vi "IsoSPI without MCU Spying Tool IHM.vi"() -> ()   [LabVIEW 2020]
uses:
  <vilib>/Instr/_visa.llb/VISA Flush IO Buffer Mask.ctl
  <vilib>/Utility/config.llb/Read Key (Double).vi
  Variables globales outil isospi sans MCU.vi
  <vilib>/Utility/config.llb/Read Key (U32).vi
  <vilib>/Instr/_visa.llb/VISA Configure Serial Port (Instr).vi
  <vilib>/Utility/config.llb/NI_LVConfig.lvlib
panel:
  in  "stop":bool
  out "SumOfCellsVoltage":string[][](table)
  out "LTC6811 Temperatures":string[][](table)
  out "NTC Temperatures":string[][](table)
  out "Cell Voltages":string[][](table)
  out "String from arduino":string
  in  "VISA resource 2":refnum<visa-resource-name>
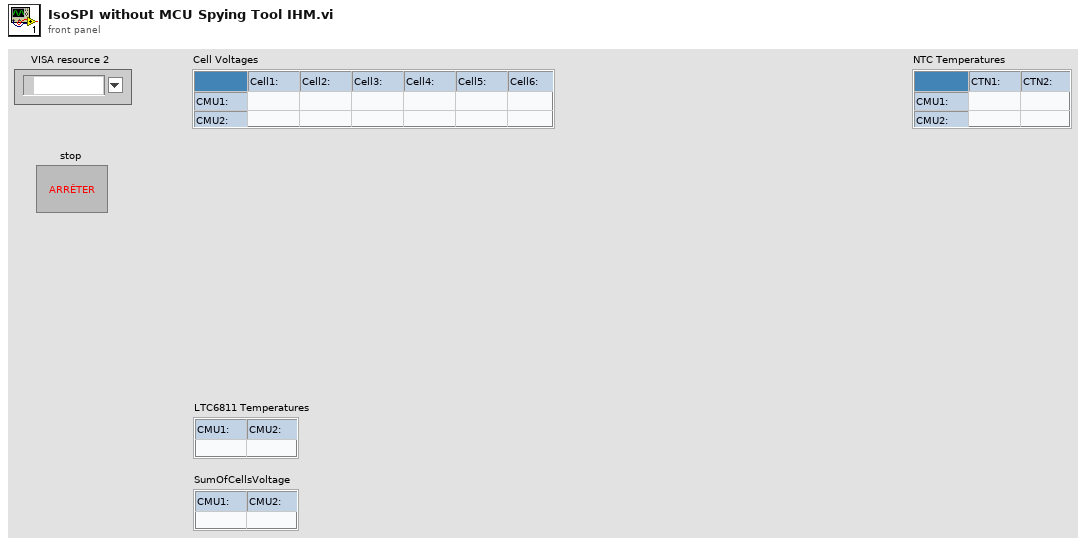
[diagram p1: front panel]
types:
  T1 = typedef "NI_LVConfig.lvlib/Config Data RefNum.ctl" = refnum<k1>
  T2 = typedef "VISA Flush IO Buffer Mask.ctl" = u16
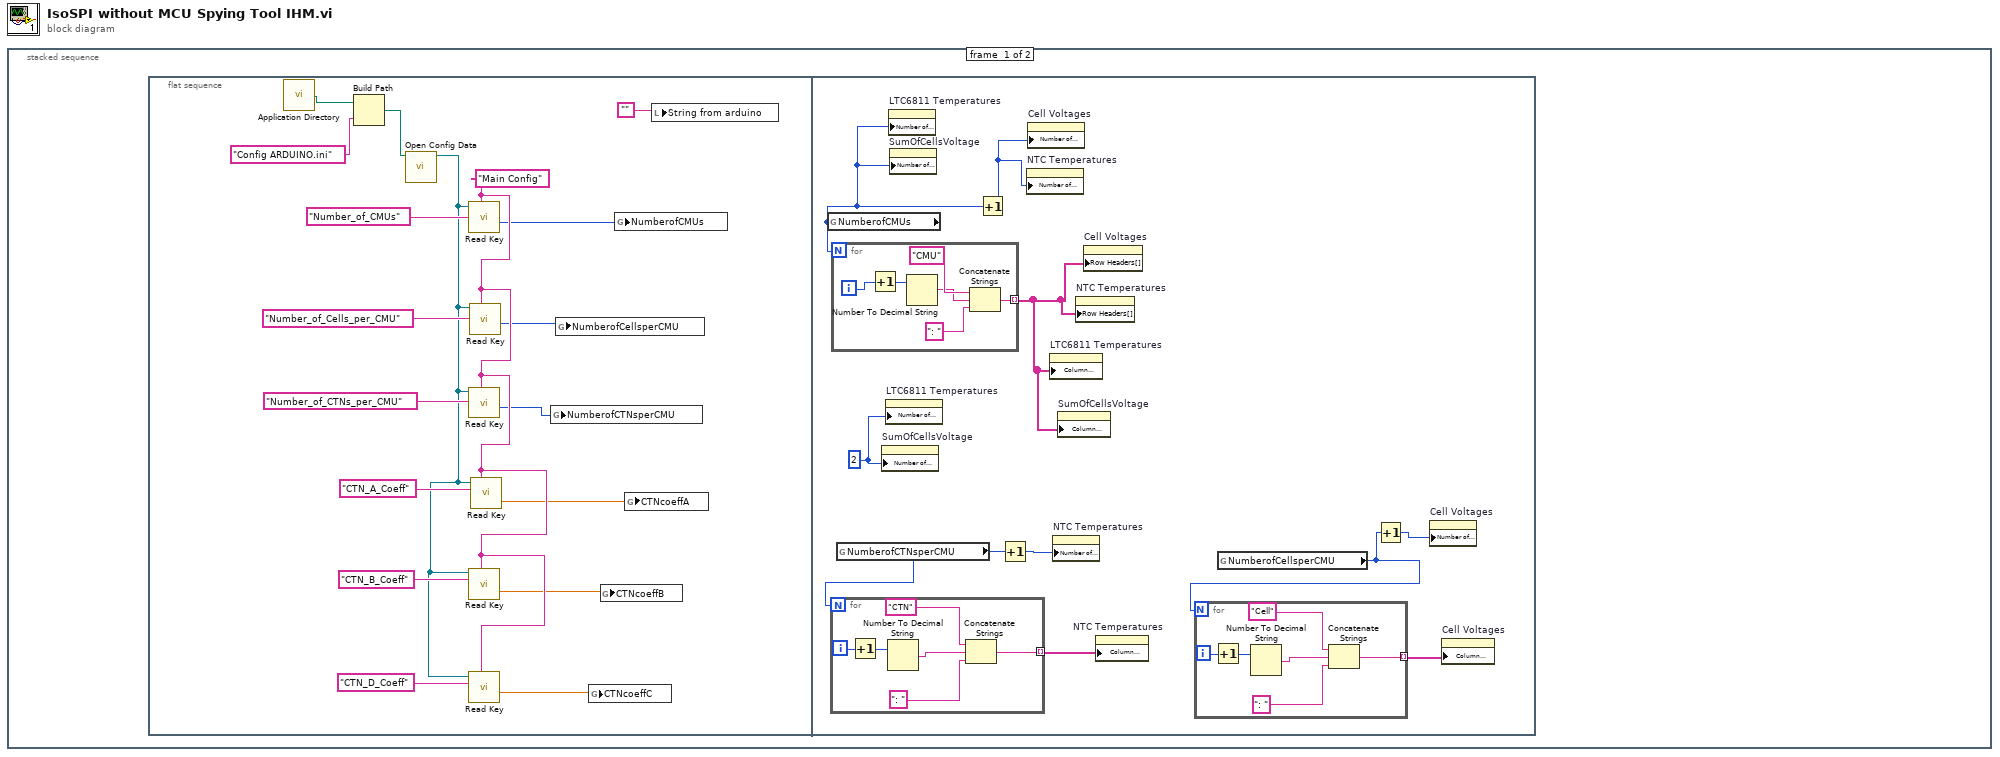
[diagram p0: block diagram]
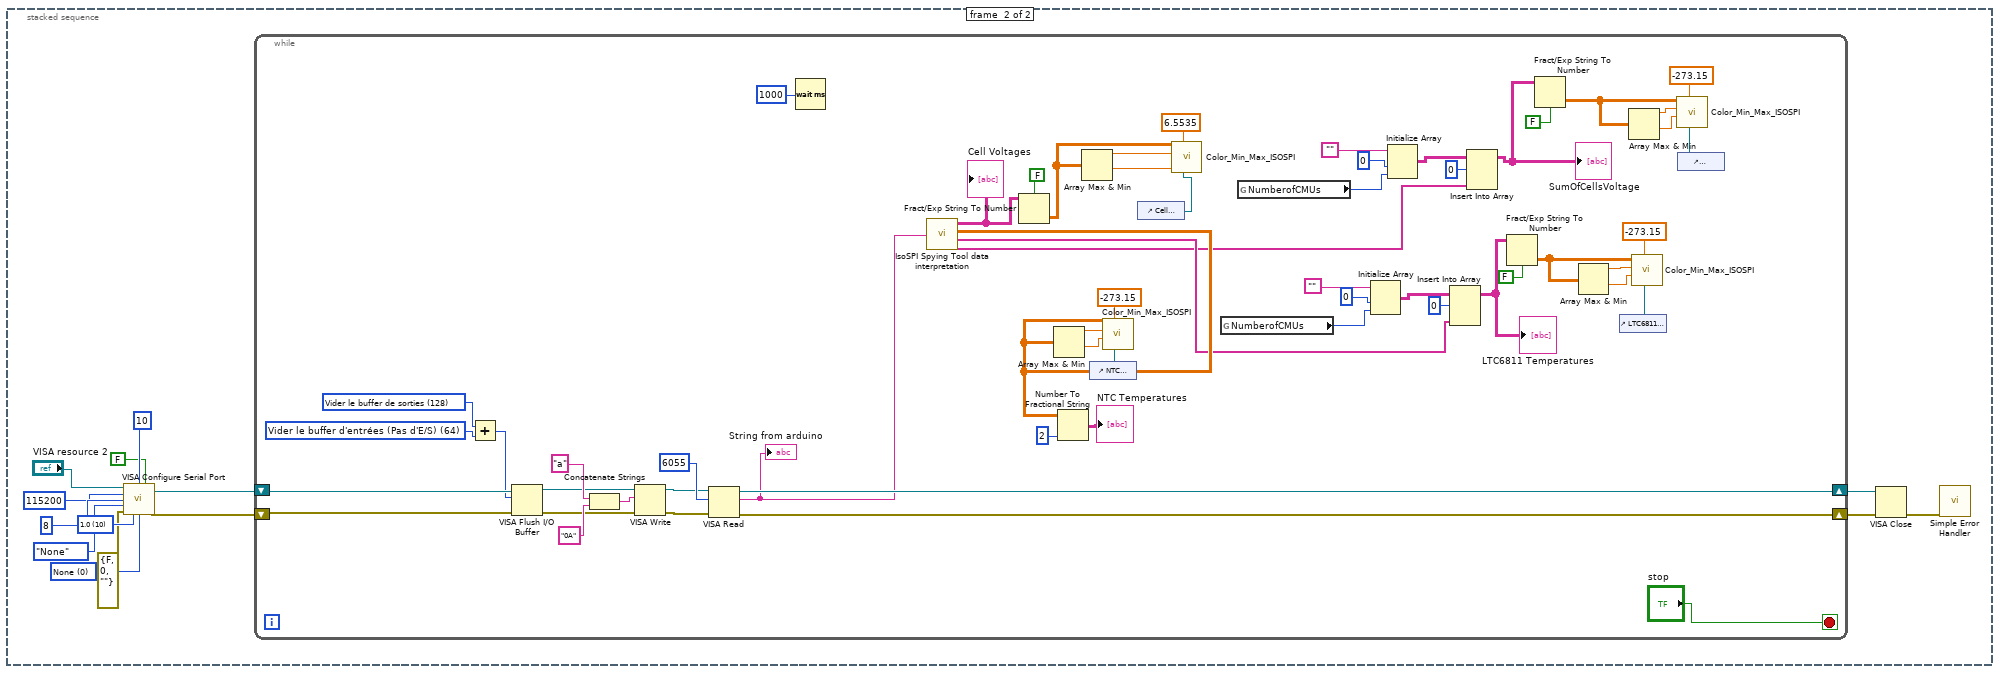
[diagram p2: hidden frame]
diagram:
  n1 = stacked-sequence {
    frame #0 {
      n2 = flat-sequence {
        frame #0 {
          w8 = "Main Config" ("section")
          n3 = call <vilib>:"Application Directory.vi"() -> ("Application Directory"=w18:path)
          n4 = Build Path(base path=w18, name or relative path="Config ARDUINO.ini") -> (appended path=w16:path)
          n5 = call <vilib>:"Open Config Data.vi"("configuration file path"=w16) -> ("refnum"=w9:T1)  [unwired: 8 in, 2 out]
          n6 = call-poly <vilib>:"Read Key.vi"("section"=w8, "key"="Number_of_CMUs", "refnum"=w9) -> ("value"=w7:u32)  [unwired: 5 in, 3 out]
          n7 = call-poly <vilib>:"Read Key.vi"("section"=w8, "key"="Number_of_CTNs_per_CMU", "refnum"=w9) -> ("value"=w5:u32)  [unwired: 5 in, 3 out]
          n8 = call-poly <vilib>:"Read Key.vi"("section"=w8, "key"="CTN_B_Coeff", "refnum"=w9) -> ("value"=w3:dbl)  [unwired: 5 in, 3 out]
          n9 = call-poly <vilib>:"Read Key.vi"("section"=w8, "key"="CTN_D_Coeff", "refnum"=w9) -> ("value"=w2:dbl)  [unwired: 5 in, 3 out]
          n10 = call-poly <vilib>:"Read Key.vi"("section"=w8, "key"="Number_of_Cells_per_CMU", "refnum"=w9) -> ("value"=w6:u32)  [unwired: 5 in, 3 out]
          n11 = call-poly <vilib>:"Read Key.vi"("section"=w8, "key"="CTN_A_Coeff", "refnum"=w9) -> ("value"=w4:dbl)  [unwired: 5 in, 3 out]
          n12 = global write "Variables globales outil isospi sans MCU.vi" "NumberofCTNsperCMU"(w5) -> ()
          n13 = global write "Variables globales outil isospi sans MCU.vi" "NumberofCellsperCMU"(w6) -> ()
          n14 = global write "Variables globales outil isospi sans MCU.vi" "CTNcoeffC"(w2) -> ()
          n15 = global write "Variables globales outil isospi sans MCU.vi" "CTNcoeffB"(w3) -> ()
          n16 = global write "Variables globales outil isospi sans MCU.vi" "NumberofCMUs"(w7) -> ()
          n17 = global write "Variables globales outil isospi sans MCU.vi" "CTNcoeffA"(w4) -> ()
          n18 = local write "String from arduino"("") -> ()
        }
        frame #1 {
          w20 = u32 2 ("Nombre de lignes")
          n19 = global read "Variables globales outil isospi sans MCU.vi" "NumberofCMUs"() -> (w19:u32)
          n20 = for {
            N: w19 -> [_]
            tunnel: [w41] -> w21 mode=indexing
            i -> [w46]
            n21 = Increment(x=w46) -> (x+1=w45:i32)
            n22 = Number To Decimal String(number=w45) -> (decimal integer string=w43:string)  [unwired: 1 in]
            n23 = Concatenate Strings("CMU", w43, ": ") -> (w41:string)
          }
          n24 = global read "Variables globales outil isospi sans MCU.vi" "NumberofCTNsperCMU"() -> (w24:u32)
          n25 = for {
            N: w24 -> [_]
            tunnel: [w29] -> w23 mode=indexing
            i -> [w34]
            n26 = Increment(x=w34) -> (x+1=w33:i32)
            n27 = Number To Decimal String(number=w33) -> (decimal integer string=w32:string)  [unwired: 1 in]
            n28 = Concatenate Strings("CTN", w32, ": ") -> (w29:string)
          }
          n29 = property on="SumOfCellsVoltage" class="Tbl (strict)"("Number of Rows"=w20) -> ()  [unwired: 2 in, 2 out]
          n30 = property on="LTC6811 Temperatures" class="Tbl (strict)"("Number of Rows"=w20) -> ()  [unwired: 2 in, 2 out]
          n31 = property on="LTC6811 Temperatures" class="Tbl (strict)"("Number of Columns"=w19) -> ()  [unwired: 2 in, 2 out]
          n32 = property on="SumOfCellsVoltage" class="Tbl (strict)"("Number of Columns"=w19) -> ()  [unwired: 2 in, 2 out]
          n33 = Increment(x=w19) -> (x+1=w22:u32)
          n34 = Increment(x=w24) -> (x+1=w25:u32)
          n35 = property on="NTC Temperatures" class="Tbl (strict)"("Number of Rows"=w22) -> ()  [unwired: 2 in, 2 out]
          n36 = property on="Cell Voltages" class="Tbl (strict)"("Number of Rows"=w22) -> ()  [unwired: 2 in, 2 out]
          n37 = property on="LTC6811 Temperatures" class="Tbl (strict)"("Column Headers[]"=w21) -> ()  [unwired: 2 in, 2 out]
          n38 = property on="NTC Temperatures" class="Tbl (strict)"("Number of Columns"=w25) -> ()  [unwired: 2 in, 2 out]
          n39 = property on="SumOfCellsVoltage" class="Tbl (strict)"("Column Headers[]"=w21) -> ()  [unwired: 2 in, 2 out]
          n40 = property on="NTC Temperatures" class="Tbl (strict)"("Row Headers[]"=w21) -> ()  [unwired: 2 in, 2 out]
          n41 = property on="Cell Voltages" class="Tbl (strict)"("Row Headers[]"=w21) -> ()  [unwired: 2 in, 2 out]
          n42 = property on="NTC Temperatures" class="Tbl (strict)"("Column Headers[]"=w23) -> ()  [unwired: 2 in, 2 out]
          n43 = global read "Variables globales outil isospi sans MCU.vi" "NumberofCellsperCMU"() -> (w27:u32)
          n44 = for {
            N: w27 -> [_]
            tunnel: [w35] -> w28 mode=indexing
            i -> [w40]
            n45 = Increment(x=w40) -> (x+1=w39:i32)
            n46 = Number To Decimal String(number=w39) -> (decimal integer string=w38:string)  [unwired: 1 in]
            n47 = Concatenate Strings("Cell", w38, ": ") -> (w35:string)
          }
          n48 = Increment(x=w27) -> (x+1=w26:u32)
          n49 = property on="Cell Voltages" class="Tbl (strict)"("Number of Columns"=w26) -> ()  [unwired: 2 in, 2 out]
          n50 = property on="Cell Voltages" class="Tbl (strict)"("Column Headers[]"=w28) -> ()  [unwired: 2 in, 2 out]
        }
      }
    }
    frame #1 {
      w59 = u16 0 items=["None", "XON/XOFF", "RTS/CTS", "XON/XOFF & RTS/CTS", "DTR/DSR", "XON/XOFF & DTR/DSR"] ("flow control (0:none)")
      w58 = u16 10 items=["1.0"=10, "1.5"=15, "2.0"=20] ("stop bits (10: 1 bit)")
      n51 = call-poly "VISA Configure Serial Port"("VISA resource name"="VISA resource 2", "termination char\n(0xA = '\\n' = LF)"=u8 10 ("termination char\n(0xA = '\\n' = LF)"), "Enable Termination\nChar (T)"=FALSE ("Enable Termination\nChar (T)"), "baud rate (9600)"=u32 115200, "data bits (8)"=u16 8, "parity (0:none)"=enum16{"None", "Odd", "Even", "Mark", "Space"}."None", "error in (no error)"=errorcluster {"status"=FALSE, "code"=0, "source"=""}, "stop bits (10: 1 bit)"=w58, "flow control (0:none)"=w59) -> ("VISA resource name out"=w48:refnum<visa-resource-name>, "error out"=w47:errorcluster)  [unwired: 5 in]
      n52 = while {
        shift-right: [w118] -> w50
        shift-left: w48 -> [w116]
        shift-right: [w117] -> w49
        shift-left: w47 -> [w115]
        stop <- "stop" stop-if-true
        w62 = T2 64 items=["Vider le buffer d'entrées"=16, "Écrire le buffer de sorties sur le périphérique"=32, "Vider le buffer d'entrées (Pas d'E/S)"=64, "Vider le buffer de sorties"=128] ("Mask")
        w63 = T2 128 items=["Vider le buffer d'entrées"=16, "Écrire le buffer de sorties sur le périphérique"=32, "Vider le buffer d'entrées (Pas d'E/S)"=64, "Vider le buffer de sorties"=128] ("Mask")
        n53 = Add(x=w63, y=w62) -> (x+y=w61:T2)
        n54 = VISA Flush I/O Buffer(VISA resource name=w116, mask (16)=w61, error in (no error)=w115) -> (VISA resource name out=w65:refnum<visa-resource-name>, error out=w64:errorcluster)
        n55 = Concatenate Strings("a" ("buffer d'écriture"), "0A" ("chaîne")) -> (w68:string)
        n56 = VISA Write(VISA resource name=w65, write buffer=w68, error in (no error)=w64) -> (VISA resource name out=w69:refnum<visa-resource-name>, error out=w70:errorcluster)  [unwired: 1 out]
        n57 = VISA Read(VISA resource name=w69, byte count=u32 6055 ("nombre d'octets"), error in (no error)=w70) -> (VISA resource name out=w118:refnum<visa-resource-name>, read buffer=w114:string, error out=w117:errorcluster)  [unwired: 1 out]
        "String from arduino" <- w114
        n58 = Wait (ms)(milliseconds to wait=u32 1000 ("attente (ms)")) -> ()  [unwired: 1 out]
        n59 = call "IsoSPI Spying Tool data interpretation.vi"("String from arduino"=w114) -> ("Cell voltages"=w111:string[][], "NTC Temperatures"=w102:dbl[][], "LTC6811 Temperatures"=w93:string[], "SumOfCellsVoltage"=w87:string[])
        "Cell Voltages" <- w111
        n60 = Fract/Exp String To Number(use system decimal point (T)=FALSE ("utiliser le séparateur décimal du système (V)"), string=w111) -> (number=w108:dbl[][])  [unwired: 2 in, 1 out]
        n61 = Array Max & Min(array=w102) -> (max value=w101:dbl, min value=w100:dbl)  [unwired: 2 out]
        n62 = Number To Fractional String(number=w102, precision (6)=i16 2 ("précision (6)")) -> (F-format string=→"NTC Temperatures":string[][])  [unwired: 2 in]
        n63 = Array Max & Min(array=w108) -> (max value=w107:dbl, min value=w106:dbl)  [unwired: 2 out]
        n64 = control-ref of="NTC Temperatures"() -> (w104:refnum<vi>)
        n65 = call "Color_Min_Max_ISOSPI.vi"("Table en entrée"=w104, "valeur invalide"=-273.15, "valeur min"=w100, "valeur max"=w101, "Tableau"=w102) -> ()  [unwired: 2 in]
        n66 = control-ref of="Cell Voltages"() -> (w109:refnum<vi>)
        n67 = call "Color_Min_Max_ISOSPI.vi"("Table en entrée"=w109, "valeur invalide"=6.5535, "valeur min"=w106, "valeur max"=w107, "Tableau"=w108) -> ()  [unwired: 2 in]
        n68 = global read "Variables globales outil isospi sans MCU.vi" "NumberofCMUs"() -> (w96:u32)
        n69 = global read "Variables globales outil isospi sans MCU.vi" "NumberofCMUs"() -> (w90:u32)
        n70 = Initialize Array("", 0 ("taille de la dimension"), w96) -> (w95:string[][])
        n71 = Initialize Array("", 0 ("taille de la dimension"), w90) -> (w91:string[][])
        n72 = Insert Into Array(array=w95, index (row)=0 ("indice (ligne)"), new element=w93) -> (w85:string[][])  [unwired: 1 in]
        "LTC6811 Temperatures" <- w85
        n73 = Insert Into Array(array=w91, index (row)=0 ("indice (ligne)"), new element=w87) -> (w77:string[][])  [unwired: 1 in]
        "SumOfCellsVoltage" <- w77
        n74 = Fract/Exp String To Number(use system decimal point (T)=FALSE ("utiliser le séparateur décimal du système (V)"), string=w85) -> (number=w84:dbl[][])  [unwired: 2 in, 1 out]
        n75 = Fract/Exp String To Number(use system decimal point (T)=FALSE ("utiliser le séparateur décimal du système (V)"), string=w77) -> (number=w76:dbl[][])  [unwired: 2 in, 1 out]
        n76 = Array Max & Min(array=w84) -> (max value=w83:dbl, min value=w82:dbl)  [unwired: 2 out]
        n77 = control-ref of="LTC6811 Temperatures"() -> (w86:refnum<vi>)
        n78 = Array Max & Min(array=w76) -> (max value=w80:dbl, min value=w81:dbl)  [unwired: 2 out]
        n79 = call "Color_Min_Max_ISOSPI.vi"("Table en entrée"=w86, "valeur invalide"=-273.15, "valeur min"=w82, "valeur max"=w83, "Tableau"=w84) -> ()  [unwired: 2 in]
        n80 = control-ref of="SumOfCellsVoltage"() -> (w78:refnum<vi>)
        n81 = call "Color_Min_Max_ISOSPI.vi"("Table en entrée"=w78, "valeur invalide"=-273.15, "valeur min"=w81, "valeur max"=w80, "Tableau"=w76) -> ()  [unwired: 2 in]
      }
      n82 = VISA Close(VISA resource name=w50, error in (no error)=w49) -> (error out=w51:errorcluster)
      n83 = call <vilib>:"Simple Error Handler.vi"("error in (no error)"=w51) -> ()  [unwired: 4 in, 5 out]
    }
  }
